vi "DjtgSetAuxReset.vi"(8 "Error In":errorcluster, 9 "Reset Pin Enable":bool, 10 "Reset Pin Value":bool, 11 "Device Number":u32) -> (0 "Error Out":errorcluster, 3 "Device Number":u32)   [LabVIEW 2011, in "LVH-Adept.lvlib" / "DJTG.lvlib"]
doc: "This function is used to set the AUX RESET pin to the specified state. A boolean TRUE value causes the pin to be set to the logic 1 state and a FALSE value causes the pin to be set to the logic 0 state. Specifying a boolean FALSE for fEnOutput disables output on the AUX RESET pin. JTAG interface pins to the specified states. This function is not supported unless the dprpJtgSetAuxReset bit is set in the port properties for the port."
uses:
  DJTG.lvlib
  Private/Type Defs/Error.ctl
  djtg.dll
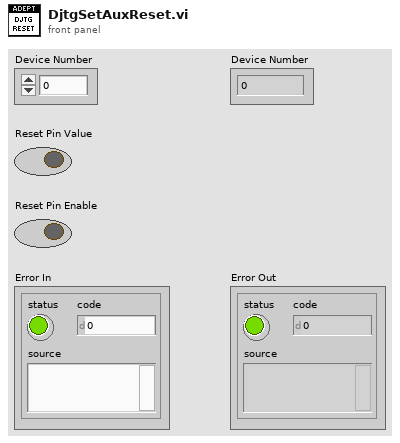
[diagram p1: front panel]
types:
  T1 = typedef "LVH-Adept.lvlib/DJTG.lvlib/Error.ctl" = enum16{"Unknown", "Enable", "PutTmsTdiBits", "GetTdoBits", "Disable", "Close", "Set Aux Reset", "Port Properties", "Get Speed", "Set Speed", "Get Port Count", "Get Batch Properties", "Enable Port", "Set Tmd Tdi Tck", "Get Tms Tdi Tdo Tck", "Put Tdi Bits", "Put Tms Bits", "Clock Tck", "Wait", "Batch", "Flash FPGA"}
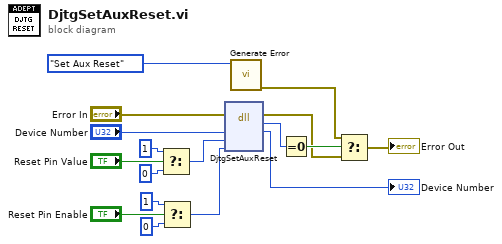
[diagram p0: block diagram]
diagram:
  n1 = Select(t=u8 1, s="Reset Pin Value", f=u8 0) -> (s? t:f=w3:u8)
  n2 = Select(t=u8 1, s="Reset Pin Enable", f=u8 0) -> (s? t:f=w2:u8)
  n3 = dll-call lib="djtg.dll" fn="DjtgSetAuxReset"(error in="Error In", "HIF"="Device Number", "fReset"=w3, "fEnOutput"=w2) -> (error out=w13:errorcluster, "Success"=w15:u32, "HIF"=→"Device Number":u32)  [unwired: 4 in, 1 out]
  n4 = call "Generate Error.vi"("DJTG Error"=Error."Set Aux Reset") -> ("Error Out"=w14:errorcluster)  [unwired: 10 in]
  n5 = Equal To 0?(x=w15) -> (x = 0?=w16:bool)
  n6 = Select(t=w14, s=w16, f=w13) -> (s? t:f=→"Error Out":errorcluster)
